vi "getHeaveConf.vi"(8 "error in (no error)":errorcluster, 11 "pHandle":u32) -> (0 "error out":errorcluster, 3 "return type":i32)   [LabVIEW 2011, in "sbgLabView.lvlib"]
uses:
  sbgLabView.lvlib
  sbgMatLab.dll
panel:
  out "heaveEnabled":bool
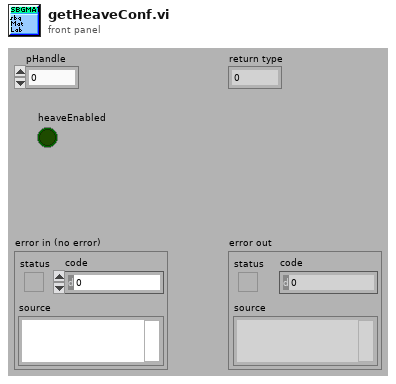
[diagram p1: front panel]
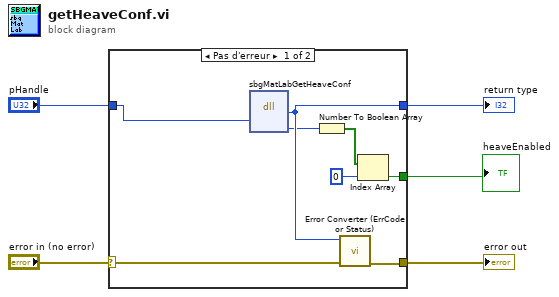
[diagram p0: block diagram]
diagram:
  n1 = case shown="Pas d'erreur" "error in (no error)" {
    selector: "error in (no error)" -> [w11 w14]
    tunnel: [w10 w14] -> w4
    tunnel: [w13 _] -> w3
    tunnel: "pHandle" -> [w12 _]
    tunnel: [w7 _] -> w1
    frame No Error {
      n2 = dll-call lib="C:/SBG-Systems/remote/projects/software/projects/labviewExample/sbgLabView/sbgMatLab.*" fn="sbgMatLabGetHeaveConf" ("sbgMatLab.dll:sbgMatLabSetMagneticDeclination")("pHandle"=w12) -> ("return type"=w13:i32, "pEnableHeave"=w9:u8)  [unwired: 5 in, 2 out]
      n3 = Number To Boolean Array(number=w9) -> (Boolean array=w8:bool[])
      n4 = call "Error Converter (ErrCode or Status).vi"("error in (no error)"=w11, "error code"=w13) -> ("error out"=w10:errorcluster)  [unwired: 9 in]
      n5 = Index Array(array=w8, index=0) -> (element=w7:bool)
    }
    frame Error {
    }
  }
  "return type" <- w3
  "error out" <- w4
  "heaveEnabled" <- w1
